vi "Handle Specific DAQ Errors.vi"(8 "error in (no error)":errorcluster, 10 "Error In":string, 11 "code":i32) -> (0 "error out":errorcluster, 3 "Error Message":string, 5 "Alert User?":bool)   [LabVIEW 2015]
doc: "This VI implements a moving average filter for this particular channel"
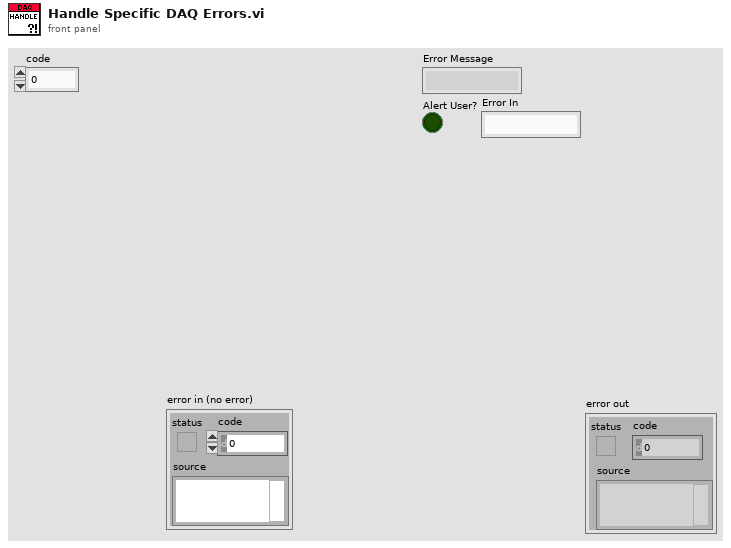
[diagram p1: front panel]
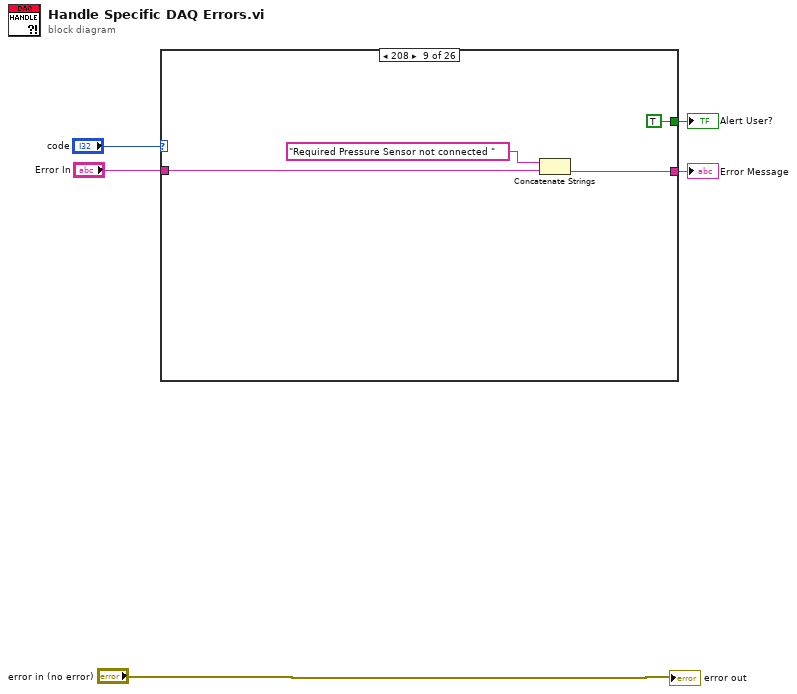
[diagram p0: block diagram]
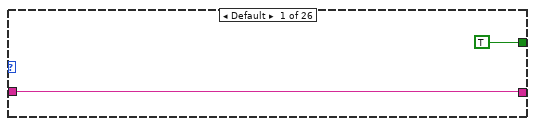
[diagram p2: hidden frame]
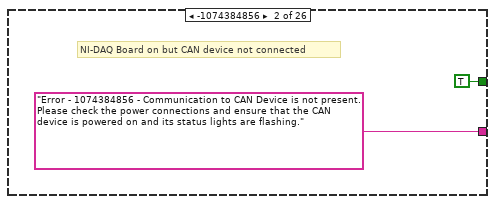
[diagram p3: hidden frame]
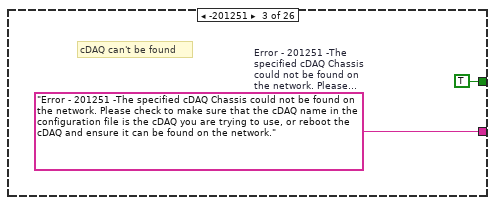
[diagram p4: hidden frame]
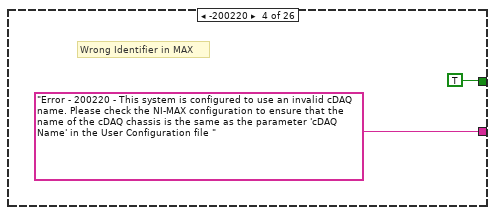
[diagram p5: hidden frame]
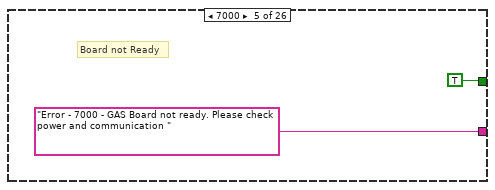
[diagram p6: hidden frame]
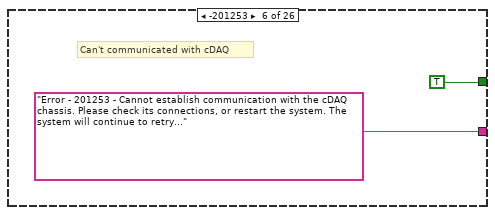
[diagram p7: hidden frame]
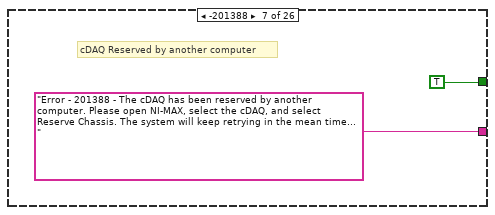
[diagram p8: hidden frame]
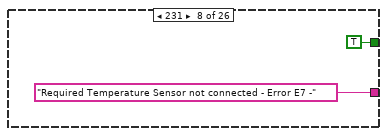
[diagram p9: hidden frame]
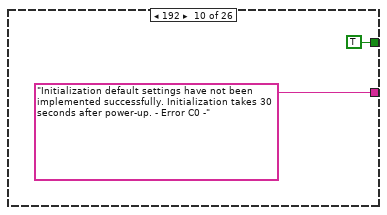
[diagram p10: hidden frame]
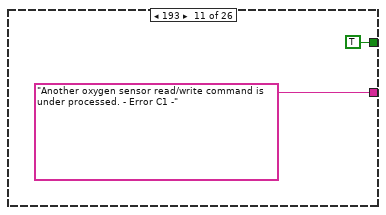
[diagram p11: hidden frame]
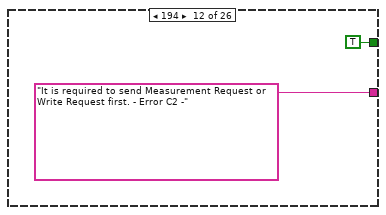
[diagram p12: hidden frame]
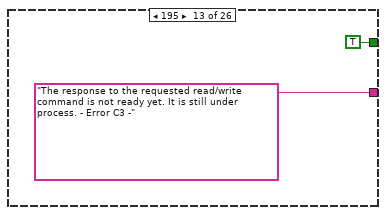
[diagram p13: hidden frame]
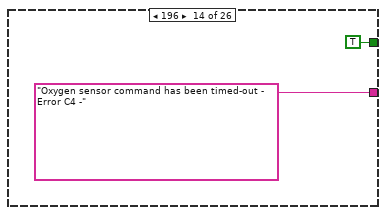
[diagram p14: hidden frame]
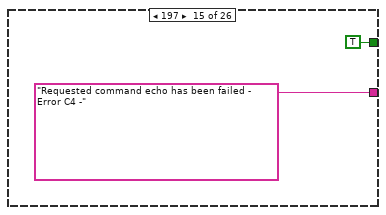
[diagram p15: hidden frame]
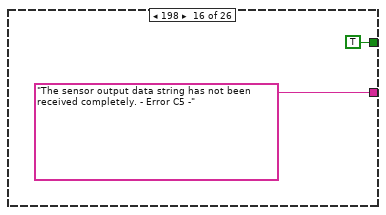
[diagram p16: hidden frame]
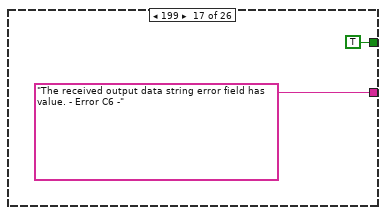
[diagram p17: hidden frame]
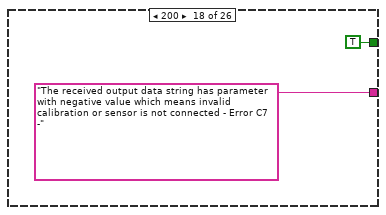
[diagram p18: hidden frame]
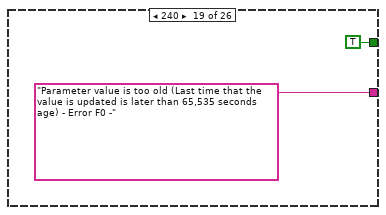
[diagram p19: hidden frame]
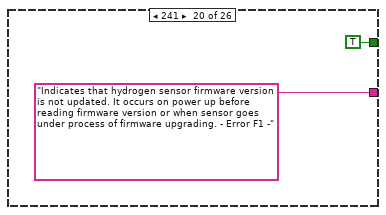
[diagram p20: hidden frame]
diagram:
  n1 = case shown="208" "code" {
    tunnel: [w6 "Error - 1074384856 - Communication to CAN Device is not present. Please check the power connections and ensure that the CAN device is powered on and its status lights are flashing." w11 "Error - 200220 - This system is configured to use an invalid cDAQ name. Please check the NI-MAX configuration to ensure that the name of the cDAQ chassis is the same as the parameter 'cDAQ Name' in the User Configuration file " "Error - 7000 - GAS Board not ready. Please check power and communication " "Error - 201253 - Cannot establish communication with the cDAQ chassis. Please check its connections, or restart the system. The system will continue to retry..." "Error - 201388 - The cDAQ has been reserved by another computer. Please open NI-MAX, select the cDAQ, and select Reserve Chassis. The system will keep retrying in the mean time... " "Required Temperature Sensor not connected - Error E7 -" ("Error In") w22 "Initialization default settings have not been implemented successfully. Initialization takes 30 seconds after power-up. - Error C0 -" ("Error In") "Another oxygen sensor read/write command is under processed. - Error C1 -" ("Error In") "It is required to send Measurement Request or Write Request first. - Error C2 -" ("Error In") "The response to the requested read/write command is not ready yet. It is still under process. - Error C3 -" ("Error In") "Oxygen sensor command has been timed-out - Error C4 -" ("Error In") "Requested command echo has been failed - Error C4 -" ("Error In") "The sensor output data string has not been received completely. - Error C5 -" ("Error In") "The received output data string error field has value. - Error C6 -" ("Error In") "The received output data string has parameter with negative value which means invalid calibration or sensor is not connected - Error C7 -" ("Error In") "Parameter value is too old (Last time that the value is updated is later than 65,535 seconds age) - Error F0 -" ("Error In") "Indicates that hydrogen sensor firmware version is not updated. It occurs on power up before reading firmware version or when sensor goes under process of firmware upgrading. - Error F1 -" ("Error In") "Indicates that sensor is active in wrong interface (Modbus/CLI) to implement CAN request. - Error F2 -" ("Error In") "This error is received when a CAN request in CLI is sent while another request is under process or sensor is not ready to accept the request. For instance, sending hex bytes before sending firmware upgrade initialization command.  - Error F3 -" ("Error In") "A buffer with size of 96 bytes is allocated to store received bytes from CAN. The error is occurred when buffer is full. Upon receiving the error, the CAN command should be sent again.  - Error F4 -" ("Error In") "The error is occurred when hydrogen sensor is already under resetting (power cycle) process. - Error F5 -" ("Error In") "Error - 201003 - The physical channel does not exist. Please check the modules within the cDAQ chassis, or edit the global virtual channel configuration in NI-MAX" _] -> w3
    tunnel: [TRUE TRUE TRUE TRUE TRUE TRUE TRUE TRUE TRUE TRUE TRUE TRUE TRUE TRUE TRUE TRUE TRUE TRUE TRUE TRUE TRUE TRUE TRUE TRUE TRUE FALSE] -> w2
    tunnel: "Error In" -> [w6 _ _ _ _ _ _ _ w24 _ _ _ _ _ _ _ _ _ _ _ _ _ _ _ _ _]
    frame Default {
    }
    frame -1074384856 {
      # "NI-DAQ Board on but CAN device not connected"
    }
    frame -201251 {
      w11 = "Error - 201251 -The specified cDAQ Chassis could not be found on the network. Please check to make sure that the cDAQ name in the configuration file is the cDAQ you are trying to use, or reboot the cDAQ and ensure it can be found on the network."  # Error - 201251 -The specified cDAQ Chassis could not be found on the network. Please check to make sure that the cDAQ name in the configuration file is the cDAQ you are trying to use, or reboot the cDAQ and ensure it can be found on the network.
      # "cDAQ can't be found"
    }
    frame -200220 {
      # "Wrong Identifier in MAX"
    }
    frame 7000 {
      # "Board not Ready"
    }
    frame -201253 {
      # "Can't communicated with cDAQ"
    }
    frame -201388 {
      # "cDAQ Reserved by another computer"
    }
    frame 231 {
    }
    frame 208 {
      n2 = Concatenate Strings("Required Pressure Sensor not connected " ("Error In"), w24) -> (w22:string)
    }
    frame 192 {
    }
    frame 193 {
    }
    frame 194 {
    }
    frame 195 {
    }
    frame 196 {
    }
    frame 197 {
    }
    frame 198 {
    }
    frame 199 {
    }
    frame 200 {
    }
    frame 240 {
    }
    frame 241 {
    }
    frame 242 {
    }
    frame 243 {
    }
    frame 244 {
    }
    frame 245 {
    }
    frame -201003 {
      # "Module not plugged in"
    }
    frame -201550 {
      # "Timed out, just ignore this error"
    }
  }
  "Error Message" <- w3
  "Alert User?" <- w2
  "error out" <- "error in (no error)"
